vi "Set cif_manager_QuerySystemStatusResponse.vi"(7 "Complete Call (T)":bool=TRUE, 8 "error in (no error)":errorcluster, 10 "package_templatemessage":T1, 11 "gRPCid":T6) -> (0 "error out":errorcluster)   [LabVIEW 2021, in "CIF_Manager_server.lvlib"]
uses:
  CIF_Manager_server.lvlib
  <vilib>/gRPC/LabVIEW gRPC Library/Shared/grpcId.ctl
  cif_manager_QuerySystemStatusResponse.ctl
  cif_manager_SystemStatus.ctl
  cif_manager_ClockConversionArray.ctl
  cif_manager_ClockConversion.ctl
  cif_manager_TimePair.ctl
  cif_manager_QuerySystemStatusResponse_Flat.ctl
  cif_manager_SystemStatus_Flat.ctl
  cif_manager_ClockConversionArray_Flat.ctl
  cif_manager_ClockConversion_Flat.ctl
  cif_manager_TimePair_Flat.ctl
  dcc74a39-081a-4bdd-860b-8ed792803c96.vi
  <vilib>/gRPC/LabVIEW gRPC Library/Shared/TranslateGrpcError.vi
  RichToFlatcif_manager_SystemStatus.vi
  RichToFlatcif_manager_ClockConversionArray.vi
  RichToFlatcif_manager_ClockConversion.vi
  RichToFlatcif_manager_TimePair.vi
  <vilib>/gRPC/LabVIEW gRPC Library/Server API/Server/Get Server DLL Path.vi
  <vilib>/Utility/error.llb/Error Cluster From Error Code.vi
  <vilib>/gRPC/LabVIEW gRPC Library/grpc-lvsupport-release.lvlib
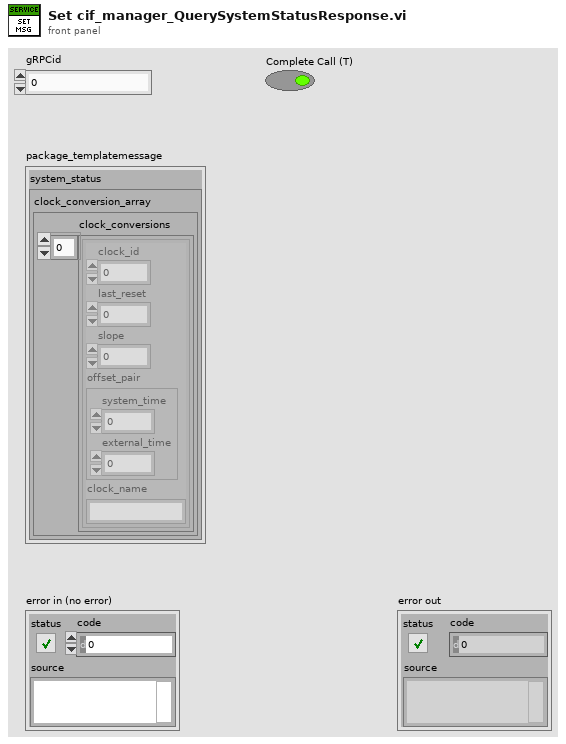
[diagram p1: front panel]
types:
  T1 = typedef "CIF_Manager_server.lvlib/cif_manager_QuerySystemStatusResponse.ctl" = cluster{"system_status":T2}
  T2 = typedef "CIF_Manager_server.lvlib/cif_manager_SystemStatus.ctl" = cluster{"clock_conversion_array":T3}
  T3 = typedef "CIF_Manager_server.lvlib/cif_manager_ClockConversionArray.ctl" = cluster{"clock_conversions":T4[]}
  T4 = typedef "CIF_Manager_server.lvlib/cif_manager_ClockConversion.ctl" = cluster{"clock_id":u32, "last_reset":i64, "slope":dbl, "offset_pair":T5, "clock_name":string}
  T5 = typedef "CIF_Manager_server.lvlib/cif_manager_TimePair.ctl" = cluster{"system_time":i64, "external_time":i64}
  T6 = typedef "grpc-lvsupport-release.lvlib/grpcId.ctl" = u64
  T7 = typedef "CIF_Manager_server.lvlib/cif_manager_QuerySystemStatusResponse_Flat.ctl" = cluster{"system_status":T8}
  T8 = typedef "CIF_Manager_server.lvlib/cif_manager_SystemStatus_Flat.ctl" = cluster{"clock_conversion_array":T9}
  T9 = typedef "CIF_Manager_server.lvlib/cif_manager_ClockConversionArray_Flat.ctl" = cluster{"clock_conversions":T10[]}
  T10 = typedef "CIF_Manager_server.lvlib/cif_manager_ClockConversion_Flat.ctl" = cluster{"clock_id":u32, "last_reset":i64, "slope":dbl, "offset_pair":T11, "clock_name":string}
  T11 = typedef "CIF_Manager_server.lvlib/cif_manager_TimePair_Flat.ctl" = cluster{"system_time":i64, "external_time":i64}
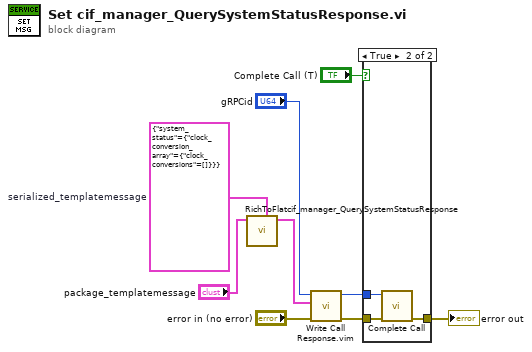
[diagram p0: block diagram]
diagram:
  w2 = T7 {"system_status"={"clock_conversion_array"={"clock_conversions"=[]}}}  # serialized_templatemessage
  n1 = call "RichToFlatcif_manager_QuerySystemStatusResponse.vi"("OutputClusterType"=w2, "InputCluster"="package_templatemessage") -> ("OutputCluster"=w1:T7)  [unwired: 9 in]
  n2 = call "Write Call Response.vim"("error in"="error in (no error)", "Response Data"=w1, "gRPCid in"="gRPCid") -> ("error out"=w6:errorcluster, "gRPCid out"=w7:T6)  [unwired: 7 in]
  n3 = case shown="True" "Complete Call (T)" {
    tunnel: [w10 w13] -> w9
    tunnel: w7 -> [_ w12]
    tunnel: w6 -> [w10 w11]
    frame False {
    }
    frame True {
      n4 = call <vilib>:"Complete Call.vi"("gRPCid"=w12, "error in"=w11) -> ("error out"=w13:errorcluster)  [unwired: 8 in]
    }
  }
  "error out" <- w9
